vi "Write Tree Control Ref.vi"(8 "error in (no error)":errorcluster, 10 "Tag Tree Reference":refnum<vi>, 11 "Process Tree View Model in":refnum<class "Process Tree View Model.lvclass">) -> (0 "error out":errorcluster, 3 "Process Tree View Model out":refnum<class "Process Tree View Model.lvclass">)   [LabVIEW 2020, in "Process Tree View Model.lvclass"]
uses:
  Process Tree View Model.lvclass
  Process Tree View Model.lvclass/Process Tree View Model.ctl
  Tree Helpers/Tag Tree/Tag Tree.lvclass
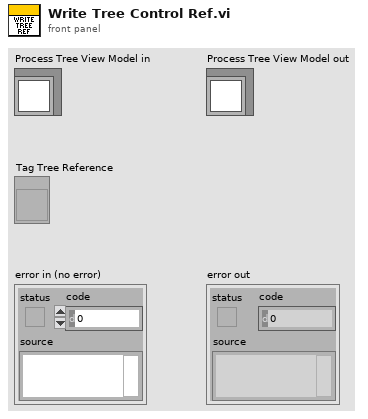
[diagram p1: front panel]
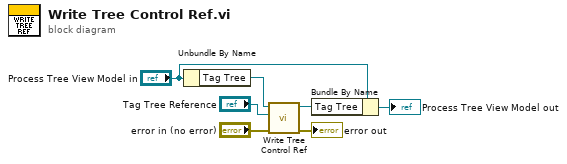
[diagram p0: block diagram]
diagram:
  n1 = Unbundle By Name("Process Tree View Model in") -> ("Tag Tree"=w6:refnum<class "Tag Tree.lvclass">)
  n2 = call "Write Tree Control Ref.vi"("error in (no error)"="error in (no error)", "Tag Tree Reference"="Tag Tree Reference", "Tag Tree In"=w6) -> ("error out"=→"error out":errorcluster, "Tag Tree Out"=w3:refnum<class "Tag Tree.lvclass">)  [unwired: 7 in]
  n3 = Bundle By Name(cluster="Process Tree View Model in", "Tag Tree"=w3) -> (→"Process Tree View Model out":refnum<class "Process Tree View Model.lvclass">)
